vi "Initialize Host Serial Port.vi"(0 "VISA In":refnum<visa-resource-name>, 5 "baud rate (9600)":u32=9600, 7 "SerPort Config":T1={"termChar"=10, "timeout"=10000, "baud"=9600, "data bits"=8, "parity"=enum."None", "stop bits"=10, "flow control (0:none)"=0} {"flow control (0:none)" items=["None", "XON/XOFF", "RTS/CTS", "XON/XOFF & RTS/CTS", "DTR/DSR", "XON/XOFF & DTR/DSR"]; "stop bits" items=["1.0"=10, "1.5"=15, "2.0"=20]; "data bits" min=5 max=8 step=1; "termChar" format="%.0x"}, 11 "error in (no error)":errorcluster) -> (4 "VISA Out":refnum<visa-resource-name>, 6 "semaphore out":T2, 15 "error out":errorcluster)   [LabVIEW 2020]
doc: "Developed by Kevin Thompson\nkevin@thompsonengineering.net\n\nCopyright 2018-2020\nThompson Engineering, LLC\nInitializes the VISA Serial Port for the WATLOW device connected on 'VISAIn' I/O address. In case of error, it will not perform the operation and pass out the error.\n==============================\nNOTE: <baud rate> control input overrides value from <SerPort Config> control."
uses:
  SerialPort Config--cluster.ctl
  <vilib>/Instr/_visa.llb/VISA Configure Serial Port (Instr).vi
panel:
  in  "EnableTermChar":bool
  # "NOTE: <baud rate> control\ninput overrides value from\n<SerPort Config> control."
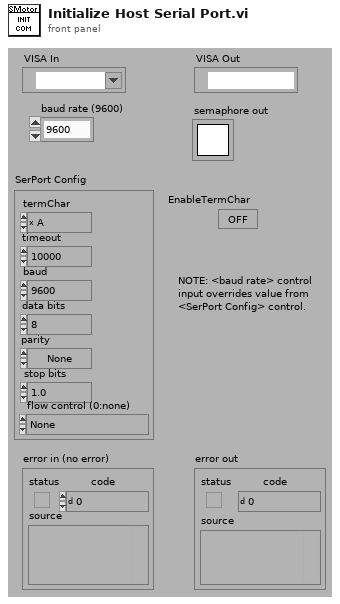
[diagram p1: front panel]
types:
  T1 = typedef "SerialPort Config--cluster.ctl" = cluster{"termChar":u8, "timeout":u32, "baud":u32, "data bits":u16, "parity":enum16{"None", "Odd", "Even", "Mark", "Space"}, "stop bits":u16, "flow control (0:none)":u16}
  T2 = typedef "Semaphore RefNum" = refnum<k1>
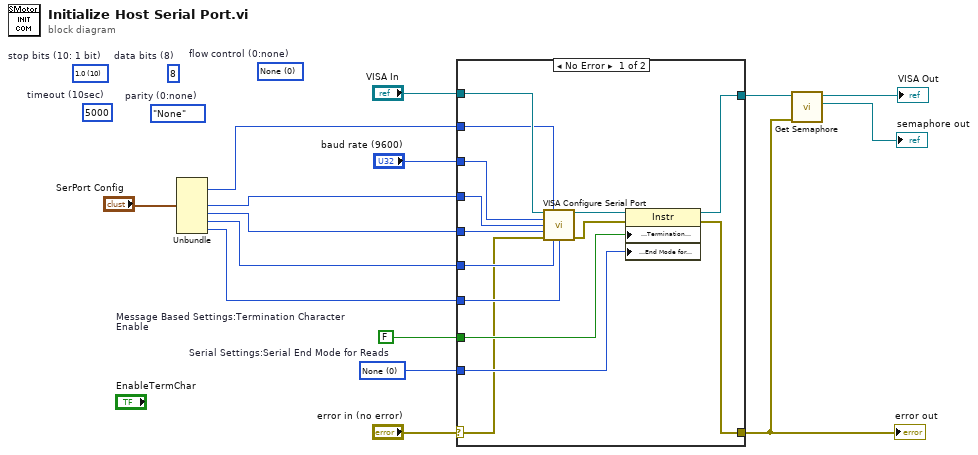
[diagram p0: block diagram]
diagram:
  w12 = u16 0 items=["None", "LastBit", "TermChar"]  # Serial Settings:Serial End Mode for Reads
  w13 = FALSE  # Message Based Settings:Termination Character Enable
  (unwired) u16 0 items=["None"=0, "XON/XOFF"=1, "RTS/CTS"=2, "DTR/DSR"=4]  # flow control (0:none)
  (unwired) u16 10 items=["1.0"=10, "1.5"=15, "2.0"=20]  # stop bits (10: 1 bit)
  (unwired) enum16{"None", "Odd", "Even", "Mark", "Space"}."None"  # parity (0:none)
  (unwired) u16 8  # data bits (8)
  (unwired) u32 5000  # timeout (10sec)
  n1 = Unbundle("SerPort Config") -> ("timeout"=w5:u32, "data bits"=w4:u16, "parity"=w3:enum16{"None", "Odd", "Even", "Mark", "Space"}, "stop bits"=w2:u16, "flow control (0:none)"=w1:u16)  [unwired: 2 out]
  n2 = case shown="No Error" "error in (no error)" {
    selector: "error in (no error)" -> [w16 w31]
    tunnel: "VISA In" -> [w29 w30]
    tunnel: w5 -> [w27 _]
    tunnel: "baud rate (9600)" -> [w26 _]
    tunnel: w4 -> [w25 _]
    tunnel: w3 -> [w24 _]
    tunnel: w2 -> [w23 _]
    tunnel: w1 -> [w22 _]
    tunnel: w13 -> [w20 _]
    tunnel: w12 -> [w19 _]
    tunnel: [w18 w31] -> w7
    tunnel: [w17 w30] -> w10
    frame No Error {
      n3 = call-poly "VISA Configure Serial Port"("VISA resource name"=w29, "timeout (10sec)"=w27, "baud rate (9600)"=w26, "data bits (8)"=w25, "parity (0:none)"=w24, "error in (no error)"=w16, "stop bits (10: 1 bit)"=w23, "flow control (0:none)"=w22) -> ("VISA resource name out"=w28:refnum<visa-resource-name>, "error out"=w21:errorcluster)  [unwired: 6 out]
      n4 = property class="Instr"(reference=w28, error in=w21, "Message Based Settings:Termination Character Enable"=w20, "Serial Settings:End Mode for Reads"=w19) -> (reference out=w17:refnum<visa-resource-name>, error out=w18:errorcluster)
    }
    frame Error {
    }
  }
  "error out" <- w7
  n5 = call "Get Semaphore.vi"("error in"=w7, "VISA In"=w10) -> ("semaphore out"=→"semaphore out":T2, "VISA Out"=→"VISA Out":refnum<visa-resource-name>)  [unwired: 3 in, 1 out]
